vi "LTE_BW.vi"(4 "LTE BW (MHz)":dbl, 5 "CLOSE VISA":bool, 6 "SET/GET":string(combo)="GET", 8 "error in":errorcluster {"code" format="%.0x"}, 10 "Timeout":u32=3000, 11 "Session In":refnum<visa-resource-name>="GPIB0::18::INSTR") -> (0 "error out":errorcluster {"code" format="%.0x"}, 2 "INST":string, 3 "reference out":refnum<visa-resource-name>)   [LabVIEW 2018]
doc: "Launches the Instrument I/O Assistant, which you can use to communicate with message-based instruments and graphically parse the response. For example you can communicate with an instrument that uses a serial, Ethernet, or GPIB interface."
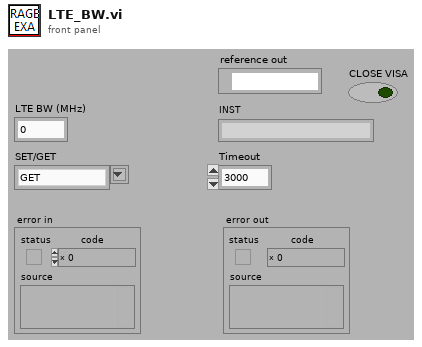
[diagram p1: front panel]
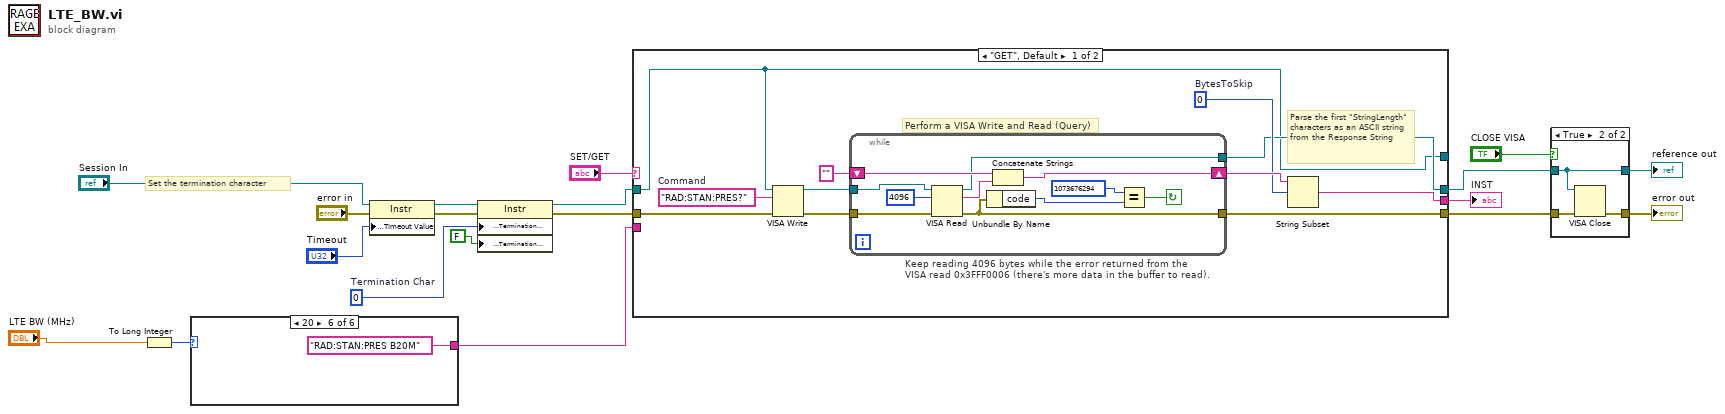
[diagram p0: block diagram]
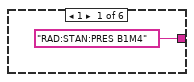
[diagram p2: hidden frame]
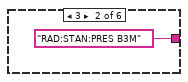
[diagram p3: hidden frame]
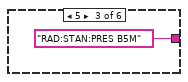
[diagram p4: hidden frame]
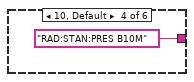
[diagram p5: hidden frame]
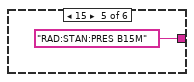
[diagram p6: hidden frame]
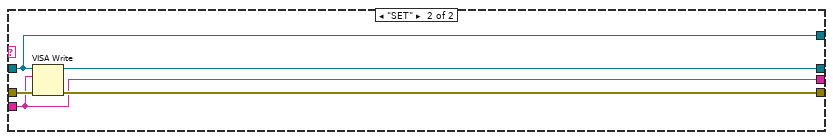
[diagram p8: hidden frame]
diagram:
  w14 = u8 0  # Termination Char
  # "Set the termination character"
  n1 = To Long Integer(number="LTE BW (MHz)") -> (32bit integer=w3:i32)
  n2 = case shown="20" w3 {
    tunnel: ["RAD:STAN:PRES B1M4" ("WRITE WFM1") "RAD:STAN:PRES B3M" ("WRITE WFM1") "RAD:STAN:PRES B5M" ("WRITE WFM1") "RAD:STAN:PRES B10M" ("WRITE WFM1") "RAD:STAN:PRES B15M" ("WRITE WFM1") "RAD:STAN:PRES B20M" ("WRITE WFM1")] -> w2
    frame 1 {
    }
    frame 3 {
    }
    frame 5 {
    }
    frame 10, Default {
    }
    frame 15 {
    }
    frame 20 {
    }
  }
  n3 = property class="Instr"(reference="Session In", error in="error in", "General Settings:Timeout Value"="Timeout") -> (reference out=w13:refnum<visa-resource-name>, error out=w16:errorcluster)
  n4 = property class="Instr"(reference=w13, error in=w16, "Message Based Settings:Termination Character"=w14, "Message Based Settings:Termination Character Enable"=FALSE ("enable")) -> (reference out=w4:refnum<visa-resource-name>, error out=w15:errorcluster)
  n5 = case shown="\"GET\", Default" "SET/GET" {
    tunnel: w15 -> [w36 w52]
    tunnel: [w33 w51] -> w9
    tunnel: [w31 w49] -> w11
    tunnel: [w26 w48] -> _
    tunnel: w2 -> [_ w49]
    tunnel: [w28 w50] -> w6
    tunnel: w4 -> [w26 w48]
    frame "GET", Default {
      w29 = 0  # BytesToSkip
      w27 = "RAD:STAN:PRES?"  # Command
      # "Parse the first \"StringLength\" characters as an ASCII string from the Response String"
      # "Perform a VISA Write and Read (Query)"
      # "Keep reading 4096 bytes while the error returned from the\nVISA read 0x3FFF0006 (there's more data in the buffer to read)."
      n6 = VISA Write(VISA resource name=w26, write buffer=w27, error in (no error)=w36) -> (VISA resource name out=w35:refnum<visa-resource-name>, error out=w34:errorcluster)  [unwired: 1 out]
      n7 = while {
        tunnel: w35 -> [w44]
        shift-right: [w38] -> w30
        shift-left: "" -> [w43]
        tunnel: w34 -> [w41]
        tunnel: [w40] -> w33
        tunnel: [w37] -> w28
        stop <- w39 continue-if-true
        n8 = VISA Read(VISA resource name=w44, byte count=u32 4096 ("byte count (0)"), error in (no error)=w41) -> (VISA resource name out=w37:refnum<visa-resource-name>, read buffer=w42:string, error out=w40:errorcluster)  [unwired: 1 out]
        n9 = Unbundle By Name(w40) -> ("code"=w46:i32)
        n10 = Concatenate Strings(w43, w42) -> (w38:string)
        n11 = Equal?(x=1073676294, y=w46) -> (x = y?=w39:bool)
      }
      n12 = String Subset(string=w30, offset (0)=w29) -> (substring=w31:string)  [unwired: 1 out]
    }
    frame "SET" {
      n13 = VISA Write(VISA resource name=w48, write buffer=w49, error in (no error)=w52) -> (VISA resource name out=w50:refnum<visa-resource-name>, error out=w51:errorcluster)  [unwired: 1 out]
    }
  }
  "INST" <- w11
  n14 = case shown="True" "CLOSE VISA" {
    tunnel: w6 -> [w53 w55]
    tunnel: w9 -> [w54 w57]
    tunnel: [w54 w56] -> w8
    tunnel: [w53 w55] -> w5
    frame False {
    }
    frame True {
      n15 = VISA Close(VISA resource name=w55, error in (no error)=w57) -> (error out=w56:errorcluster)
    }
  }
  "error out" <- w8
  "reference out" <- w5
